vi "Draw Floor.vi"(5 "Name":string="Floor") -> (1 "Scene.Object Out":refnum<vi>)   [LabVIEW 2011]
uses:
  <vilib>/Utility/miscctls.llb/LV3DPointTypeDef.ctl
  <vilib>/Utility/miscctls.llb/LVTextureCoordinateArrayTypeDef.ctl
  <vilib>/picture/3D Picture Control/NI_3D Picture Control.lvlib
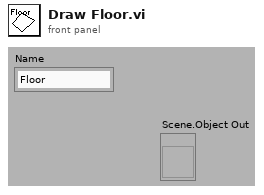
[diagram p1: front panel]
types:
  T1 = typedef "LVTextureCoordinateArrayTypeDef.ctl" = cluster{"S":sgl, "T":sgl}[]
  T2 = typedef "LV3DPointTypeDef.ctl" = cluster{"X":sgl, "Y":sgl, "Z":sgl}
  T3 = enum16{"Overall", "Per Primitive", "Per Vertex", "Binding Off"}
  T4 = enum16{"As a Decal", "With Modulation", "With Blending", "As a replacement"}
  T5 = enum16{"Points", "Lines", "Line Strip", "Line Loop", "Triangles", "Triangle Strip", "Triangle Fan", "Quads", "Quad Strip", "Polygon"}
  T6 = typedef "imagedata.ctl" = cluster{"image type":i32, "image depth":i32, "image":u8[], "mask":u8[], "colors":u32[], "Rectangle":cluster{"left":i16, "top":i16, "right":i16, "bottom":i16}}
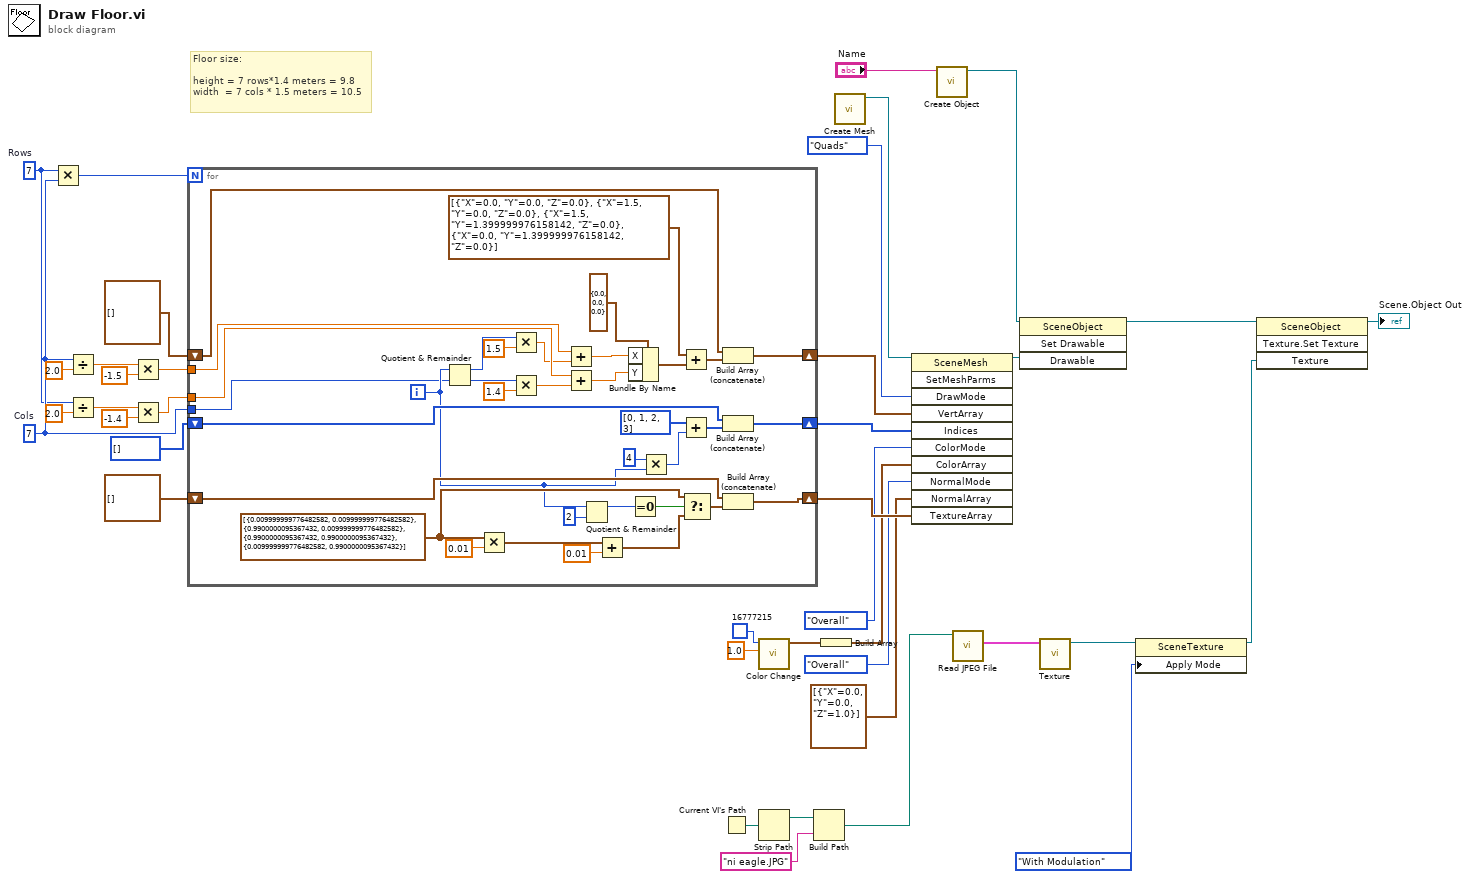
[diagram p0: block diagram]
diagram:
  w39 = 7  # Cols
  w30 = 7  # Rows
  # "Floor size:\n\nheight = 7 rows*1.4 meters = 9.8 \nwidth  = 7 cols * 1.5 meters = 10.5"
  n1 = Multiply(x=w30, y=w39) -> (x*y=w29:i32)
  n2 = Divide(x=w39, y=2.0 ("x/y")) -> (x/y=w35:dbl)
  n3 = Divide(x=w30, y=2.0 ("x/y")) -> (x/y=w33:dbl)
  n4 = Multiply(x=w35, y=-1.5) -> (x*y=w38:dbl)
  n5 = Multiply(x=w33, y=-1.4) -> (x*y=w37:dbl)
  n6 = for {
    N: w29 -> [_]
    shift-right: [w74] -> w27
    shift-left: u32[] [] -> [w73]
    shift-right: [w72] -> w28
    shift-left: T2[] [] -> [w71]
    shift-right: [w69] -> w26
    shift-left: T1 [] ("Texture Coordinate Array") -> [w70]
    tunnel: w37 -> [w51]
    tunnel: w38 -> [w45]
    tunnel: w39 -> [w52]
    i -> [w53]
    w59 = T1 [{"S"=0.01, "T"=0.01}, {"S"=0.99, "T"=0.01}, {"S"=0.99, "T"=0.99}, {"S"=0.01, "T"=0.99}] ("Texture Coordinate Array")
    n7 = Quotient & Remainder(x=w53, y=w52) -> (x-y*floor(x/y)=w44:i32, floor(x/y)=w49:i32)
    n8 = Multiply(x=w59, y=0.01 ("T")) -> (x*y=w56:cluster{"S":dbl, "T":dbl}[])
    n9 = Multiply(x=w44, y=1.5) -> (x*y=w46:dbl)
    n10 = Multiply(x=w49, y=1.4) -> (x*y=w50:dbl)
    n11 = Add(x=w45, y=w46) -> (x+y=w42:dbl)
    n12 = Add(x=w51, y=w50) -> (x+y=w41:dbl)
    n13 = Quotient & Remainder(x=w53, y=2) -> (x-y*floor(x/y)=w61:i32)  [unwired: 1 out]
    n14 = Add(x=w56, y=0.01 ("T")) -> (x+y=w54:cluster{"S":dbl, "T":dbl}[])
    n15 = Bundle By Name(cluster=T2 {"X"=0.0, "Y"=0.0, "Z"=0.0} ("3D Point"), "X"=w42, "Y"=w41) -> (w40:T2)
    n16 = Equal To 0?(x=w61) -> (x = 0?=w60:bool)
    n17 = Multiply(x=4, y=w53) -> (x*y=w65:i32)
    n18 = Add(x=T2[] [{"X"=0.0, "Y"=0.0, "Z"=0.0}, {"X"=1.5, "Y"=0.0, "Z"=0.0}, {"X"=1.5, "Y"=1.4, "Z"=0.0}, {"X"=0.0, "Y"=1.4, "Z"=0.0}] ("Vertex Array"), y=w40) -> (x+y=w67:T2[])
    n19 = Add(x=u32[] [0, 1, 2, 3] ("Indices"), y=w65) -> (x+y=w63:u32[])
    n20 = Select(t=w59, s=w60, f=w54) -> (s? t:f=w57:cluster{"S":dbl, "T":dbl}[])
    n21 = Build Array (concatenate)(w71, w67) -> (w72:T2[])
    n22 = Build Array (concatenate)(w73, w63) -> (w74:u32[])
    n23 = Build Array (concatenate)(w70, w57) -> (w69:cluster{"S":dbl, "T":dbl}[])
  }
  n24 = Current VI's Path() -> (path=w8:path)
  n25 = call <vilib>:"Color Change.vi"("Alpha"=1.0, "Color"=u32 16777215) -> ("RGBA"=w21:cluster{"R":sgl, "G":sgl, "B":sgl, "A":sgl})  [unwired: 9 out]
  n26 = Strip Path(path=w8) -> (stripped path=w9:path)  [unwired: 1 out]
  n27 = Build Path(base path=w9, name or relative path="ni eagle.JPG" ("path to JPEG file")) -> (appended path=w11:path)
  n28 = Build Array(w21) -> (w22:cluster{"R":sgl, "G":sgl, "B":sgl, "A":sgl}[])
  n29 = call <vilib>:"Create Mesh.vi"() -> ("New Mesh Refnum"=w2:refnum<vi>)  [unwired: 1 in, 10 out]
  n30 = invoke class="SceneMesh" method="SetMeshParms"(reference=w2, "DrawMode"=T5."Quads" ("Draw Mode"), "VertArray"=w28, "Indices"=w27, "ColorMode"=T3."Overall" ("Color Binding Mode"), "ColorArray"=w22, "NormalMode"=T3."Overall" ("Normal Binding Mode"), "NormalArray"=T2[] [{"X"=0.0, "Y"=0.0, "Z"=1.0}] ("Normal Array"), "TextureArray"=w26) -> (reference out=w7:refnum<vi>)  [unwired: 2 in, 10 out]
  n31 = call <vilib>:"Create Object.vi"("Name"="Name") -> ("Scene:New Object"=w6:refnum<vi>)  [unwired: 1 in, 9 out]
  n32 = call <vilib>:"Read JPEG File.vi"("path to JPEG file"=w11) -> ("image data"=w12:T6)  [unwired: 1 in, 9 out]
  n33 = invoke class="SceneObject" method="Set Drawable"(reference=w6, "Drawable"=w7) -> (reference out=w1:refnum<vi>)  [unwired: 2 in, 3 out]
  n34 = call <vilib>:"Texture.vi"("Image"=w12) -> ("New Texture Refnum"=w13:refnum<vi>)  [unwired: 1 in, 9 out]
  n35 = property class="SceneTexture"(reference=w13, "Apply Mode"=T4."With Modulation") -> (reference out=w15:refnum<vi>)  [unwired: 1 in, 1 out]
  n36 = invoke class="SceneObject" method="Texture.Set Texture"(reference=w1, "Texture"=w15) -> (reference out=→"Scene.Object Out":refnum<vi>)  [unwired: 2 in, 3 out]
